vi "Read Array of Tx Frames.vi"(8 "error in":errorcluster, 11 "port node in":refnum<k20>) -> (0 "error out":errorcluster, 3 "te generic frames":refnum<k20>[](array[refnum]))   [LabVIEW 2020, in "AIM ARINC 664 Import.lvlib"]
uses:
  AIM ARINC 664 Import.lvlib
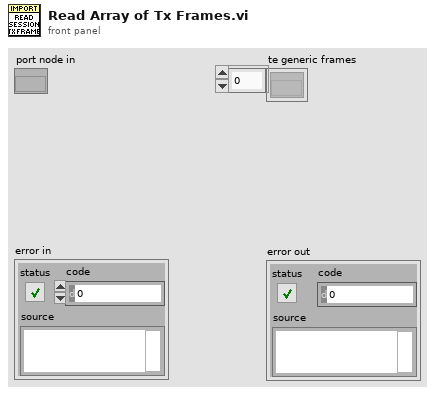
[diagram p1: front panel]
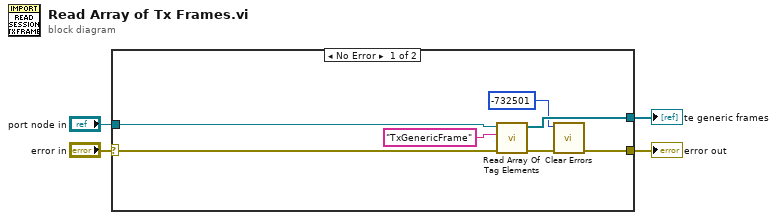
[diagram p0: block diagram]
diagram:
  n1 = case shown="No Error" "error in" {
    selector: "error in" -> [w11 w12]
    tunnel: [w8 w12] -> w4
    tunnel: "port node in" -> [w10 _]
    tunnel: [w9 _] -> w2
    frame No Error {
      n2 = call "Read Array Of Tag Elements.vi"("error in"=w11, "tag name"="TxGenericFrame", "node in"=w10) -> ("error out"=w7:errorcluster, "array of elements"=w9:refnum<k20>[])  [unwired: 7 in]
      n3 = call <vilib>:"Clear Errors.vi"("error in (no error)"=w7, "specific error code to clear (0: all)"=-732501) -> ("error out"=w8:errorcluster)  [unwired: 4 in, 1 out]
    }
    frame Error {
    }
  }
  "error out" <- w4
  "te generic frames" <- w2
